vi "$Honeywell1900 helps.vi"   [LabVIEW 2017]
uses:
  <vilib>/Utility/miscctls.llb/LVPointTypeDef.ctl
panel:
  # "扫码枪设置 by YYLL"
  # "Xenon 1900/1902"
  # "波特率默认115200"
  # "手动触发-常规模式(需要按住触发器进行读取)\n呈现模式(扫描枪在“检测到”条码后激活)下使用扫描枪。"
  # "-"
types:
  T1 = enum32{"Invalid", "Standard", "Closed", "Hidden", "Minimized", "Maximized"}
  T2 = typedef "LVPointTypeDef.ctl" = cluster{"Horizontal":i16, "Vertical":i16}
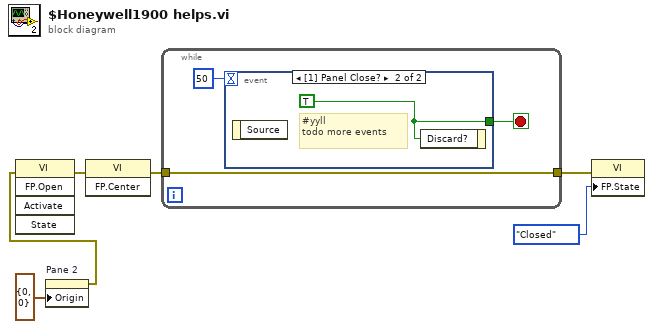
[diagram p0: block diagram]
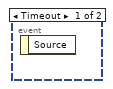
[diagram p2: hidden frame]
diagram:
  n1 = property on="Pane 2" class="Pane"("Origin"=T2 {"Horizontal"=0, "Vertical"=0}) -> (error out=w1:errorcluster)  [unwired: 2 in, 1 out]
  n2 = invoke class="VI" method="FP.Open"(error in=w1) -> (error out=w5:errorcluster)  [unwired: 4 in, 4 out]
  n3 = invoke class="VI" method="FP.Center"(error in=w5) -> (error out=w2:errorcluster)  [unwired: 2 in, 2 out]
  n4 = while {
    tunnel: [w7] -> w3
    tunnel: w2 -> [w7]
    stop <- w8 stop-if-true
    n5 = event shown="[1] Panel Close?" {
      selector: _ -> [_ _]
      dyn-events: _ -> [_ _]
      timeout: 50 -> [_ _]
      tunnel: [_ w10] -> w8
      event Timeout {
        n6 = event-data() -> ()  [unwired: 1 in, 1 out]
      }
      event Panel Close? {
        w10 = TRUE ("Discard?")
        # "#yyll\ntodo more events"
        n7 = event-data() -> ()  [unwired: 1 in, 1 out]
        n8 = event-data("Discard?"=w10) -> ()  [unwired: 1 in, 1 out]
      }
    }
  }
  n9 = property class="VI"(error in=w3, "FP.State"=T1."Closed" ("前面板窗口:状态")) -> ()  [unwired: 1 in, 2 out]
